vi "Write Channel Active.vi"(8 "error in":errorcluster, 10 "Channel Active":bool, 11 "Input Channels in":refnum<class "Input Channels.lvclass">) -> (0 "error out":errorcluster, 3 "Input Channels out":refnum<class "Input Channels.lvclass">)   [LabVIEW 2020, in "Plugin.lvlib" / "Input Channels.lvclass"]
doc: "Writes channel active."
uses:
  Input Channels.lvclass
  Input Channels.lvclass/Input Channels.ctl
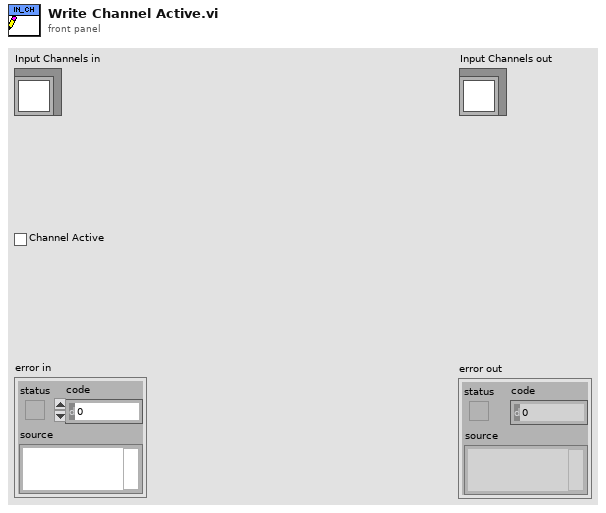
[diagram p1: front panel]
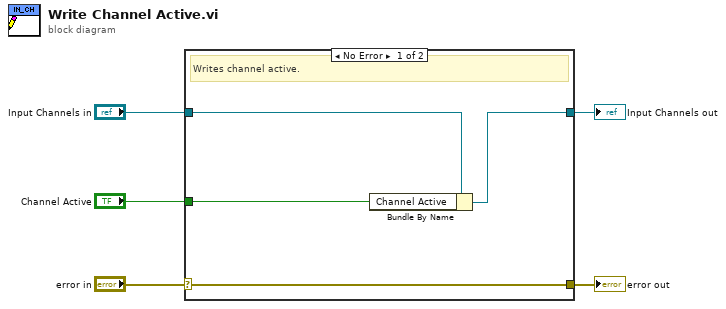
[diagram p0: block diagram]
diagram:
  n1 = case shown="No Error" "error in" {
    selector: "error in" -> [w9 w10]
    tunnel: [w9 w10] -> w4
    tunnel: [w7 w11] -> w2
    tunnel: "Input Channels in" -> [w8 w11]
    tunnel: "Channel Active" -> [w6 _]
    frame No Error {
      # "Writes channel active."
      n2 = Bundle By Name(cluster=w8, "Channel Active"=w6) -> (w7:refnum<class "Input Channels.lvclass">)
    }
    frame Error {
      # "Error"
    }
  }
  "error out" <- w4
  "Input Channels out" <- w2
